vi "MGI Bezier Inverse Multiple Solutions.vi"   [LabVIEW 2020]
doc: "Calculates bezier 0..1 parameters from y, a bezier function result. All solutions in the range 0..1 are returned, in ascending order.\n\nAuthored by David A. Moore\nsupport@mooregoodideas.com\nwww.mooregoodideas.com\n\nCopyright (c) 2010, Moore Good Ideas, Inc.\n\nAll rights reserved.\n\nRedistribution and use in source and binary forms, with or without modification, are permitted provided that the following conditions are met:\n\n * Redistributions of source code must retain the above copyright notice, this list of conditions and the following disclaimer.\n * Redistributions in binary form must reproduce the above copyright notice, this list of conditions and the following disclaimer in the documentation and/or other materials provided with the distribution.\n * Neither the name of Moore Good Ideas, Inc. nor the names of its contributors may be used to endorse or promote products derived from this software without specific prior written permission.\n\nTHIS SOFTWARE IS PROVIDED BY THE COPYRIGHT HOLDERS AND CONTRIBUTORS \"AS IS\" AND ANY EXPRESS OR IMPLIED WARRANTIES, INCLUDING, BUT NOT LIMITED TO, THE IMPLIED WARRANTIES OF MERCHANTABILITY AND FITNESS FOR A PARTICULAR PURPOSE ARE DISCLAIMED. IN NO EVENT SHALL THE COPYRIGHT OWNER OR CONTRIBUTORS BE LIABLE FOR ANY DIRECT, INDIRECT, INCIDENTAL, SPECIAL, EXEMPLARY, OR CONSEQUENTIAL DAMAGES (INCLUDING, BUT NOT LIMITED TO, PROCUREMENT OF SUBSTITUTE GOODS OR SERVICES; LOSS OF USE, DATA, OR PROFITS; OR BUSINESS INTERRUPTION) HOWEVER CAUSED AND ON ANY THEORY OF LIABILITY, WHETHER IN CONTRACT, STRICT LIABILITY, OR TORT (INCLUDING NEGLIGENCE OR OTHERWISE) ARISING IN ANY WAY OUT OF THE USE OF THIS SOFTWARE, EVEN IF ADVISED OF THE POSSIBILITY OF SUCH DAMAGE."
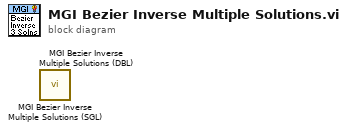
[diagram p0: block diagram]
diagram:
  n1 = call <userlib>:"MGI Bezier Inverse Multiple Solutions (SGL).vi"() -> ()  [unwired: 3 in, 1 out]
  n2 = call <userlib>:"MGI Bezier Inverse Multiple Solutions (DBL).vi"() -> ()  [unwired: 3 in, 1 out]
